vi "Read Output Till Keyword.vi"(7 "timeout [ms]":u32, 8 "error in":errorcluster, 10 "keywords":string[](array[string]), 11 "pipe in":T1) -> (0 "error out":errorcluster, 2 "read buffer":string, 3 "pipe out":T1, 5 "bytes remaining":i32)   [LabVIEW 2013, in "GOLPI library.lvlib"]
doc: "Continually reads output of GNU Octave. If one of strings specified in keywords terminal is found in output, reading stops.\nIf timeout is exceeded, returns only part of buffer and returns number of bytes remaining in the stdout buffer.\nOne of keywords should be 'error' in the case error occurs, otherwise the vi will wait till timeout."
uses:
  GOLPI library.lvlib
  LV Process.lvlibp/Pipe Handle.ctl
  LV Process.lvlibp
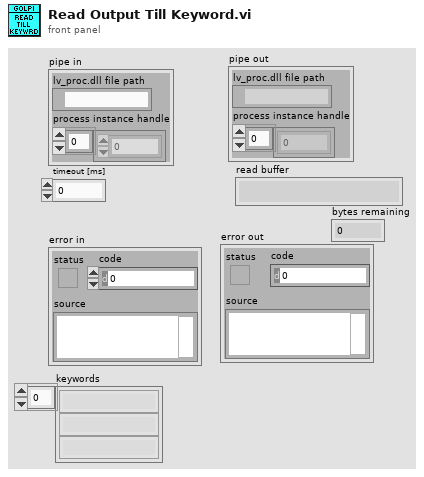
[diagram p1: front panel]
types:
  T1 = typedef "LV Process.lvlibp/Pipe Handle.ctl" = cluster{"lv_proc.dll file path":path, "process instance handle":u32[]}
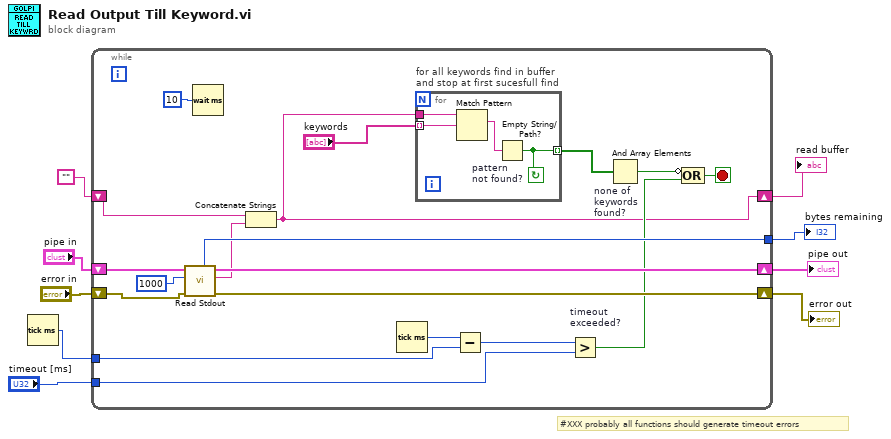
[diagram p0: block diagram]
diagram:
  # "#XXX probably all functions should generate timeout errors"
  n1 = Tick Count (ms)() -> (millisecond timer value=w1:u32)
  n2 = while {
    tunnel: [w21] -> w4
    shift-right: [w27] -> w8
    shift-left: "pipe in" -> [w28]
    shift-right: [w14] -> w5
    shift-left: "" -> [w16]
    tunnel: w1 -> [w24]
    tunnel: "timeout [ms]" -> [w22]
    shift-right: [w26] -> w7
    shift-left: "error in" -> [w25]
    stop <- w19 stop-if-true
    n3 = call "Read Stdout.vi"("error in"=w25, "byte count"=1000, "pipe in"=w28) -> ("error out"=w26:errorcluster, "read buffer"=w10:string, "pipe out"=w27:T1, "bytes remaining"=w21:i32)  [unwired: 3 in, 2 out]
    n4 = Wait (ms)(milliseconds to wait=u32 10) -> ()  [unwired: 1 out]
    n5 = Concatenate Strings(w16, w10) -> (w14:string)
    n6 = Tick Count (ms)() -> (millisecond timer value=w15:u32)
    n7 = for "for all keywords find in buffer\nand stop at first sucesfull find" {
      tunnel: w14 -> [w32]
      tunnel: "keywords" -> [w31] mode=indexing
      tunnel: [w29] -> w12 mode=indexing
      stop <- w29 continue-if-true
      n8 = Match Pattern(string=w32, regular expression=w31) -> (match substring=w30:string)  [unwired: 1 in, 3 out]
      n9 = Empty String/Path? "pattern\nnot found?"(string/path=w30) -> (empty?=w29:bool)
    }
    n10 = Subtract(x=w15, y=w24) -> (x-y=w23:u32)
    n11 = Greater? "timeout\nexceeded?"(x=w23, y=w22) -> (0:w20:bool)
    n12 = And Array Elements "none of\nkeywords\nfound?"(Boolean array=w12) -> (logical AND=w11:bool)
    n13 = Compound Arithmetic op=OR(invert w11, w20) -> (w19:bool)
  }
  "pipe out" <- w8
  "error out" <- w7
  "read buffer" <- w5
  "bytes remaining" <- w4
